vi "LTVUnicycleCtrl_Pack_Tolerance.vi"(9 "Max Heading Tolerance Rad":dbl=0.07, 10 "Max Y Tolerance M":dbl=0.03, 11 "Max X Tolerance M":dbl=0.03) -> (3 "LTV_Unicycle_Ctrl_Tolerance":T1 {"Max Y Tolerance M" format="%#_13g"; "Max X Tolerance M" format="%#_13g"; "Max Heading Tolerance Rad" format="%#_13g"})   [LabVIEW 2019, in "Trajectory_Library.lvlib"]
uses:
  Trajectory_Library.lvlib
  TypeDef/LTV_UNICYCLE_CONTROLLER_TOLERANCE.CTL
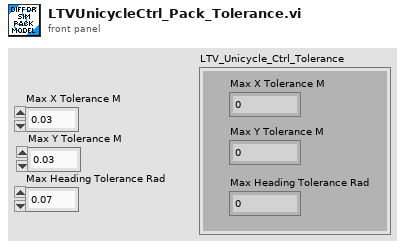
[diagram p1: front panel]
types:
  T1 = typedef "Trajectory_Library.lvlib/LTV_UNICYCLE_CONTROLLER_TOLERANCE.CTL" = cluster{"Max Heading Tolerance Rad":dbl, "Max X Tolerance M":dbl, "Max Y Tolerance M":dbl}
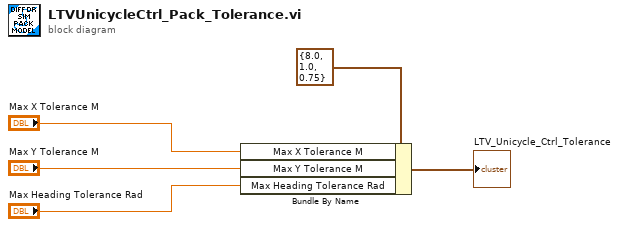
[diagram p0: block diagram]
diagram:
  n1 = Bundle By Name(cluster=T1 {"Max Heading Tolerance Rad"=8.0, "Max X Tolerance M"=1.0, "Max Y Tolerance M"=0.75} ("SngJntArmSim_Simulation _Params"), "Max X Tolerance M"="Max X Tolerance M", "Max Y Tolerance M"="Max Y Tolerance M", "Max Heading Tolerance Rad"="Max Heading Tolerance Rad") -> (→"LTV_Unicycle_Ctrl_Tolerance":T1)
